vi "3D Eval Func at Sampling Pnts.vi"(5 "Formula/VI ref":bool, 6 "VI ref":cluster{"f(x)":refnum<vi>, "data":variant}, 7 "Formula":T1, 8 "error in (no error)":errorcluster, 9 "z limit":cluster{"z lower":dbl, "z upper":dbl}={"z lower"=0.0, "z upper"=1.0}, 10 "y limit":cluster{"y lower":dbl, "y upper":dbl}={"y lower"=0.0, "y upper"=1.0}, 11 "x limit":cluster{"x lower":dbl, "x upper":dbl}={"x lower"=0.0, "x upper"=1.0}) -> (0 "error out":errorcluster, 1 "Sampling points (7-order)":dbl[][](array[numeric]), 2 "Function Evaluations (4 pts)":dbl[][][](array[numeric]), 3 "Function Evaluations (7 pts)":dbl[][][](array[numeric]))   [LabVIEW 2018, in "NI_AALPro.lvlib"]
uses:
  NI_AALPro.lvlib
  NI_Gmath.lvlib
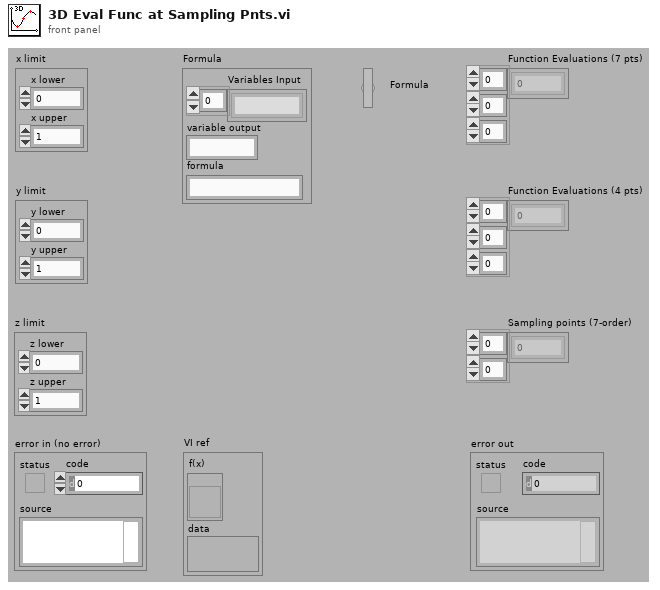
[diagram p1: front panel]
types:
  T1 = cluster{"Variables Input":string[], "variable output":string, "formula":string}
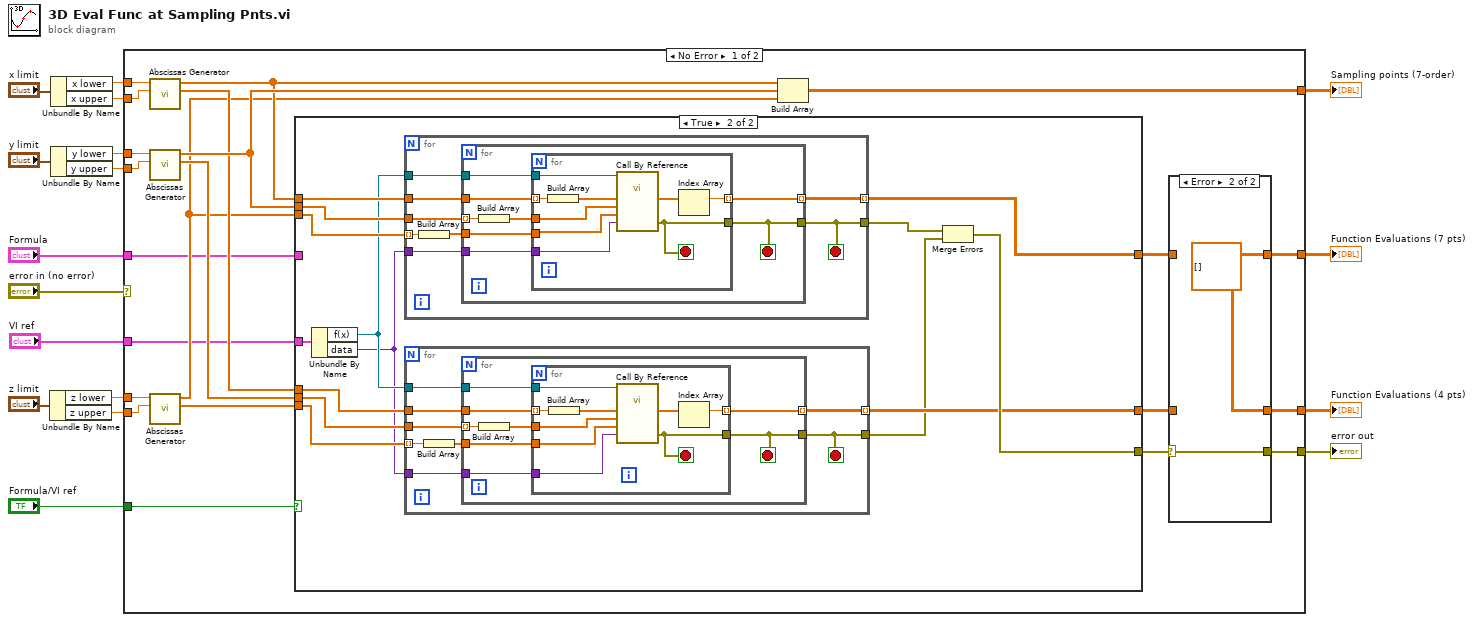
[diagram p0: block diagram]
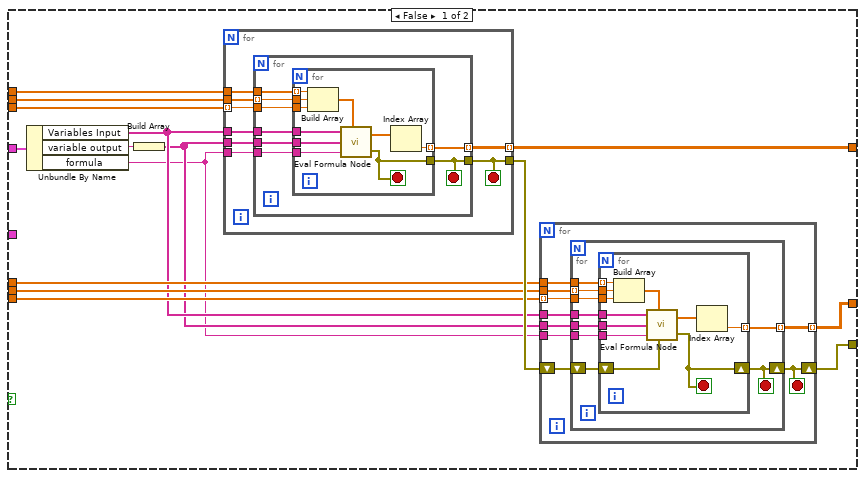
[diagram p3: hidden frame]
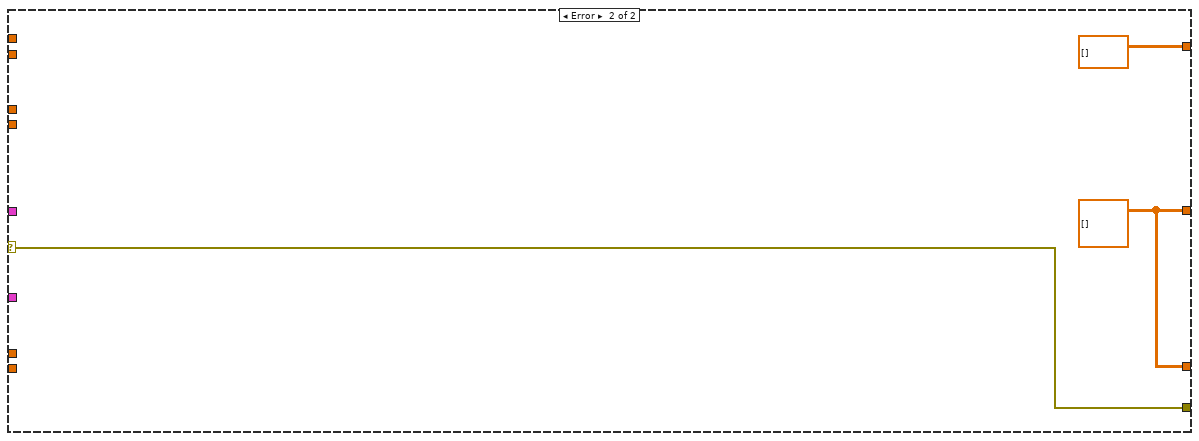
[diagram p4: hidden frame]
diagram:
  n1 = Unbundle By Name("z limit") -> ("z lower"=w5:dbl, "z upper"=w4:dbl)
  n2 = Unbundle By Name("x limit") -> ("x lower"=w12:dbl, "x upper"=w11:dbl)
  n3 = Unbundle By Name("y limit") -> ("y lower"=w9:dbl, "y upper"=w8:dbl)
  n4 = case shown="No Error" "error in (no error)" {
    selector: "error in (no error)" -> [_ w181]
    tunnel: [w33 dbl[][] []] -> w17
    tunnel: [w20 w179] -> w16
    tunnel: [w22 w181] -> w15
    tunnel: w12 -> [w39 _]
    tunnel: w11 -> [w38 _]
    tunnel: w9 -> [w37 _]
    tunnel: w8 -> [w36 _]
    tunnel: [w18 w179] -> w7
    tunnel: w5 -> [w30 _]
    tunnel: w4 -> [w29 _]
    tunnel: "Formula" -> [w26 _]
    tunnel: "VI ref" -> [w25 _]
    tunnel: "Formula/VI ref" -> [w24 _]
    frame No Error {
      n5 = call "Abscissas Generator.vi"("upper limit"=w38, "lower limit"=w39) -> ("4 points"=w32:dbl[], "7 points"=w34:dbl[])  [unwired: 8 out]
      n6 = call "Abscissas Generator.vi"("upper limit"=w36, "lower limit"=w37) -> ("4 points"=w31:dbl[], "7 points"=w35:dbl[])  [unwired: 8 out]
      n7 = call "Abscissas Generator.vi"("upper limit"=w29, "lower limit"=w30) -> ("4 points"=w28:dbl[], "7 points"=w27:dbl[])  [unwired: 8 out]
      n8 = case shown="True" w24 {
        tunnel: [w58 w119] -> w21
        tunnel: w35 -> [w57 w127]
        tunnel: w34 -> [w56 w128]
        tunnel: w32 -> [w55 w125]
        tunnel: w31 -> [w54 w124]
        tunnel: [w53 w117] -> w19
        tunnel: w28 -> [w52 w123]
        tunnel: [w51 w118] -> w23
        tunnel: w27 -> [w50 w126]
        tunnel: w26 -> [w49 _]
        tunnel: w25 -> [_ w122]
        frame False {
          n9 = Unbundle By Name(w49) -> ("Variables Input"=w48:string[], "variable output"=w47:string, "formula"=w45:string)
          n10 = Build Array(w47) -> (w46:string[])
          n11 = for {
            tunnel: [w96] -> w58 mode=indexing
            tunnel: w57 -> [w95]
            tunnel: w56 -> [w94]
            tunnel: w46 -> [w93]
            tunnel: w45 -> [w92]
            tunnel: w48 -> [w91]
            tunnel: w50 -> [w90] mode=indexing
            tunnel: [w89] -> w59
            stop <- w89 stop-if-true
            n12 = for {
              tunnel: [w104] -> w96 mode=indexing
              tunnel: w95 -> [w103] mode=indexing
              tunnel: w94 -> [w102]
              tunnel: w91 -> [w101]
              tunnel: w93 -> [w100]
              tunnel: w92 -> [w99]
              tunnel: w90 -> [w98]
              tunnel: [w97] -> w89
              stop <- w97 stop-if-true
              n13 = for {
                tunnel: w99 -> [w114]
                tunnel: w101 -> [w113]
                tunnel: w100 -> [w112]
                tunnel: w102 -> [w111] mode=indexing
                tunnel: [w110] -> w104 mode=indexing
                tunnel: w103 -> [w107]
                tunnel: w98 -> [w106]
                tunnel: [w105] -> w97
                stop <- w105 stop-if-true
                n14 = Build Array(w111, w107, w106) -> (w108:dbl[])
                n15 = call "Eval Formula Node.vi"("Variables Input"=w113, "Input Values"=w108, "Variables Output"=w112, "formula"=w114) -> ("Output Values"=w109:dbl[], "error out"=w105:errorcluster)  [unwired: 1 in]
                n16 = Index Array(array=w109) -> (element=w110:dbl)  [unwired: 1 in]
              }
            }
          }
          n17 = for {
            tunnel: w55 -> [w68]
            tunnel: w54 -> [w67]
            tunnel: w46 -> [w66]
            tunnel: w45 -> [w65]
            tunnel: [w64] -> w53 mode=indexing
            tunnel: w48 -> [w62]
            tunnel: w52 -> [w61] mode=indexing
            shift-right: [w60] -> w51
            shift-left: w59 -> [w63]
            stop <- w60 stop-if-true
            n18 = for {
              tunnel: w68 -> [w77]
              tunnel: w67 -> [w76] mode=indexing
              tunnel: w62 -> [w75]
              tunnel: w66 -> [w74]
              tunnel: w65 -> [w73]
              tunnel: [w72] -> w64 mode=indexing
              shift-right: [w69] -> w60
              shift-left: w63 -> [w71]
              tunnel: w61 -> [w70]
              stop <- w69 stop-if-true
              n19 = for {
                tunnel: w73 -> [w88]
                tunnel: w75 -> [w87]
                tunnel: w74 -> [w86]
                tunnel: w77 -> [w85] mode=indexing
                tunnel: [w84] -> w72 mode=indexing
                shift-right: [w78] -> w69
                shift-left: w71 -> [w82]
                tunnel: w76 -> [w80]
                tunnel: w70 -> [w79]
                stop <- w78 stop-if-true
                n20 = Build Array(w85, w80, w79) -> (w81:dbl[])
                n21 = call "Eval Formula Node.vi"("Variables Input"=w87, "Input Values"=w81, "Variables Output"=w86, "formula"=w88, "error in (no error)"=w82) -> ("Output Values"=w83:dbl[], "error out"=w78:errorcluster)
                n22 = Index Array(array=w83) -> (element=w84:dbl)  [unwired: 1 in]
              }
            }
          }
        }
        frame True {
          n23 = Unbundle By Name(w122) -> ("f(x)"=w121:refnum<vi>, "data"=w120:variant)
          n24 = for {
            tunnel: [w161] -> w119 mode=indexing
            tunnel: w121 -> [w160]
            tunnel: w128 -> [w159]
            tunnel: w127 -> [w158]
            tunnel: w120 -> [w157]
            tunnel: [w154] -> w115
            tunnel: w126 -> [w155] mode=indexing
            stop <- w154 stop-if-true
            n25 = Build Array(w155) -> (w156:dbl[])
            n26 = for {
              tunnel: w160 -> [w169]
              tunnel: [w162] -> w154
              tunnel: w157 -> [w168]
              tunnel: [w167] -> w161 mode=indexing
              tunnel: w159 -> [w166]
              tunnel: w158 -> [w165] mode=indexing
              tunnel: w156 -> [w163]
              stop <- w162 stop-if-true
              n27 = Build Array(w165) -> (w164:dbl[])
              n28 = for {
                tunnel: w169 -> [w178]
                tunnel: [w170] -> w162
                tunnel: w168 -> [w177]
                tunnel: [w172] -> w167 mode=indexing
                tunnel: w166 -> [w175] mode=indexing
                tunnel: w164 -> [w174]
                tunnel: w163 -> [w171]
                stop <- w170 stop-if-true
                n29 = Build Array(w175) -> (w173:dbl[])
                n30 = call-by-ref "?"(reference=w178, "data"=w177, "Z"=w171, "Y"=w174, "X"=w173) -> ("error out"=w170:errorcluster, "Array"=w176:dbl[])  [unwired: 7 in, 2 out]
                n31 = Index Array(array=w176) -> (element=w172:dbl)  [unwired: 1 in]
              }
            }
          }
          n32 = for {
            tunnel: w121 -> [w136]
            tunnel: w125 -> [w135]
            tunnel: w124 -> [w134]
            tunnel: w120 -> [w133]
            tunnel: [w132] -> w117 mode=indexing
            tunnel: [w129] -> w116
            tunnel: w123 -> [w130] mode=indexing
            stop <- w129 stop-if-true
            n33 = Build Array(w130) -> (w131:dbl[])
            n34 = for {
              tunnel: w136 -> [w144]
              tunnel: [w137] -> w129
              tunnel: w133 -> [w143]
              tunnel: [w142] -> w132 mode=indexing
              tunnel: w135 -> [w141]
              tunnel: w134 -> [w140] mode=indexing
              tunnel: w131 -> [w138]
              stop <- w137 stop-if-true
              n35 = Build Array(w140) -> (w139:dbl[])
              n36 = for {
                tunnel: w144 -> [w153]
                tunnel: [w145] -> w137
                tunnel: w143 -> [w152]
                tunnel: [w147] -> w142 mode=indexing
                tunnel: w141 -> [w150] mode=indexing
                tunnel: w139 -> [w149]
                tunnel: w138 -> [w146]
                stop <- w145 stop-if-true
                n37 = Build Array(w150) -> (w148:dbl[])
                n38 = call-by-ref "?"(reference=w153, "data"=w152, "Z"=w146, "Y"=w149, "X"=w148) -> ("error out"=w145:errorcluster, "Array"=w151:dbl[])  [unwired: 7 in, 2 out]
                n39 = Index Array(array=w151) -> (element=w147:dbl)  [unwired: 1 in]
              }
            }
          }
          n40 = Merge Errors(w115, w116) -> (w118:errorcluster)
        }
      }
      n41 = Build Array(w34, w35, w27) -> (w33:dbl[][])
      n42 = case shown="Error" w23 {
        selector: w23 -> [w42 w44]
        tunnel: [w42 w44] -> w22
        tunnel: w21 -> [w41 _]
        tunnel: [w41 w43] -> w20
        tunnel: w19 -> [w40 _]
        tunnel: [w40 w43] -> w18
        frame No Error {
        }
        frame Error {
          w43 = dbl[][][] []
        }
      }
    }
    frame Error {
      w179 = dbl[][][] []
    }
  }
  "Sampling points (7-order)" <- w17
  "Function Evaluations (7 pts)" <- w16
  "error out" <- w15
  "Function Evaluations (4 pts)" <- w7
